vi "EEI EXP7b.vi"() -> ()   [LabVIEW 2020]
panel:
  out "Array 2":dbl[][](array[numeric])
  out "Array":dbl[](array[numeric])
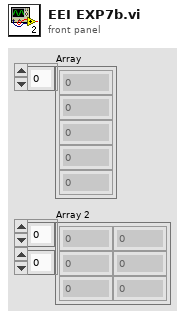
[diagram p1: front panel]
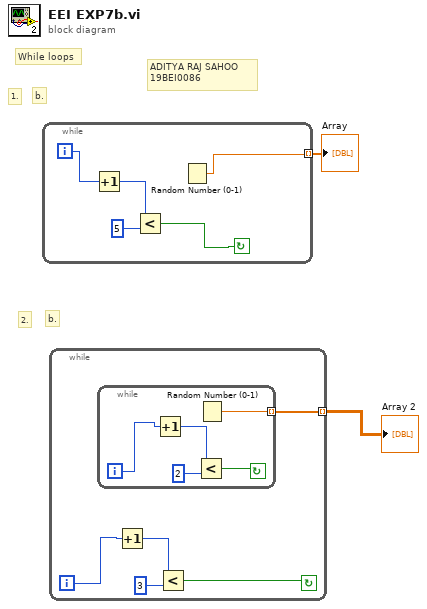
[diagram p0: block diagram]
diagram:
  # "ADITYA RAJ SAHOO\n19BEI0086"
  # "While loops"
  # "b."
  # "2."
  # "b."
  # "1."
  n1 = while {
    tunnel: [w3] -> w2 mode=indexing
    i -> [w7]
    stop <- w6 continue-if-true
    n2 = Increment(x=w7) -> (x+1=w5:i32)
    n3 = Less?(x=w5, y=5) -> (x < y?=w6:bool)
    n4 = Random Number (0-1)() -> (number: 0 to 1=w3:dbl)
  }
  "Array" <- w2
  n5 = while {
    tunnel: [w8] -> w1 mode=indexing
    i -> [w9]
    stop <- w10 continue-if-true
    n6 = while {
      tunnel: [w14] -> w8 mode=indexing
      i -> [w15]
      stop <- w13 continue-if-true
      n7 = Increment(x=w15) -> (x+1=w17:i32)
      n8 = Less?(x=w17, y=2) -> (x < y?=w13:bool)
      n9 = Random Number (0-1)() -> (number: 0 to 1=w14:dbl)
    }
    n10 = Increment(x=w9) -> (x+1=w12:i32)
    n11 = Less?(x=w12, y=3) -> (x < y?=w10:bool)
  }
  "Array 2" <- w1
